vi "parse_file.vi"(0 "File Name With Extension":string) -> (1 "command vector":T1[](array[typedef]), 2 "file_status":string)   [LabVIEW 2014]
uses:
  vi_execute.ctl
panel:
  out "error out":errorcluster
  out "File Contents":string
  out "Lines":string[](array[string])
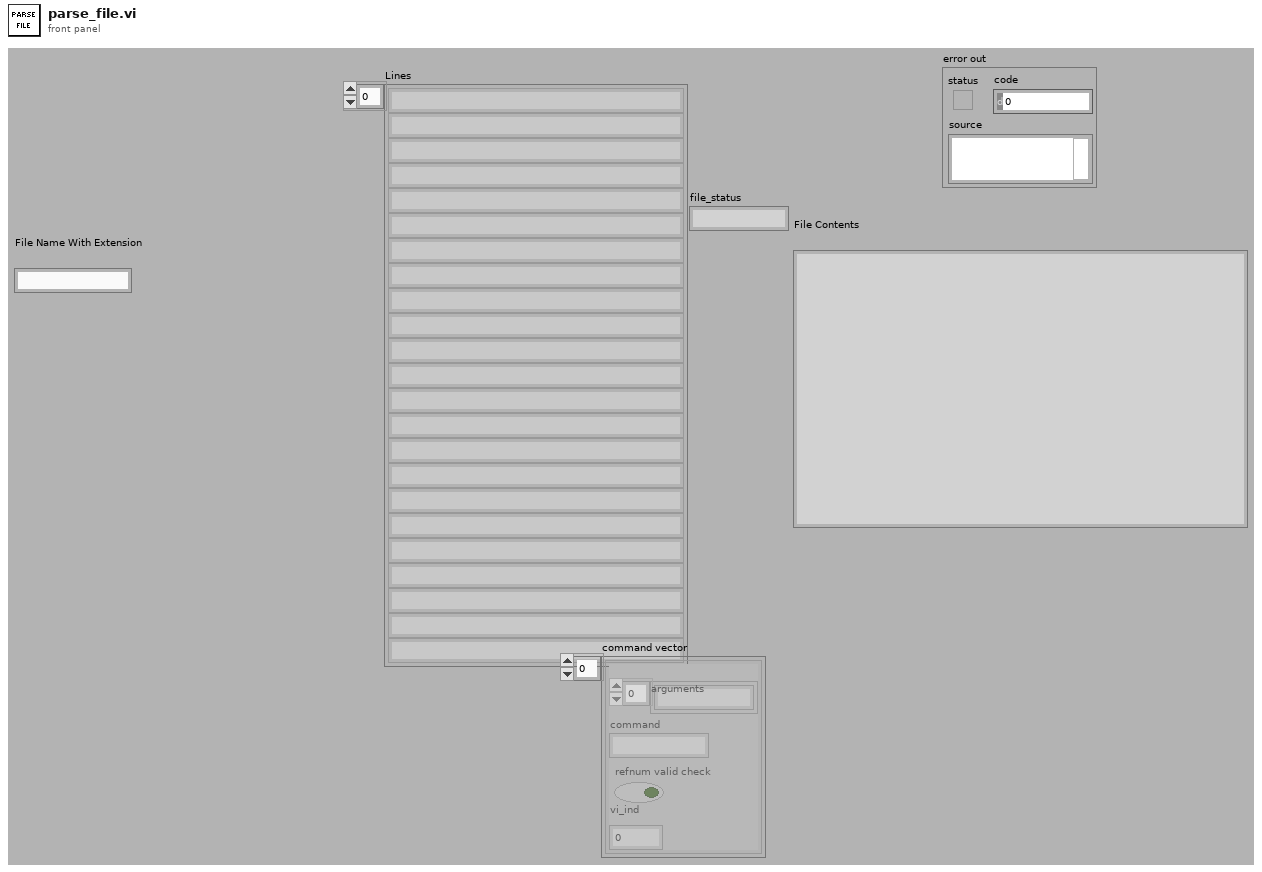
[diagram p1: front panel]
types:
  T1 = typedef "vi_execute.ctl" = cluster{"arguments":string[], "command":string, "refnum valid check":bool, "vi_ind":u8}
  T2 = cluster{"arguments":string[], "refnum name out":string, bool, "index":u8}
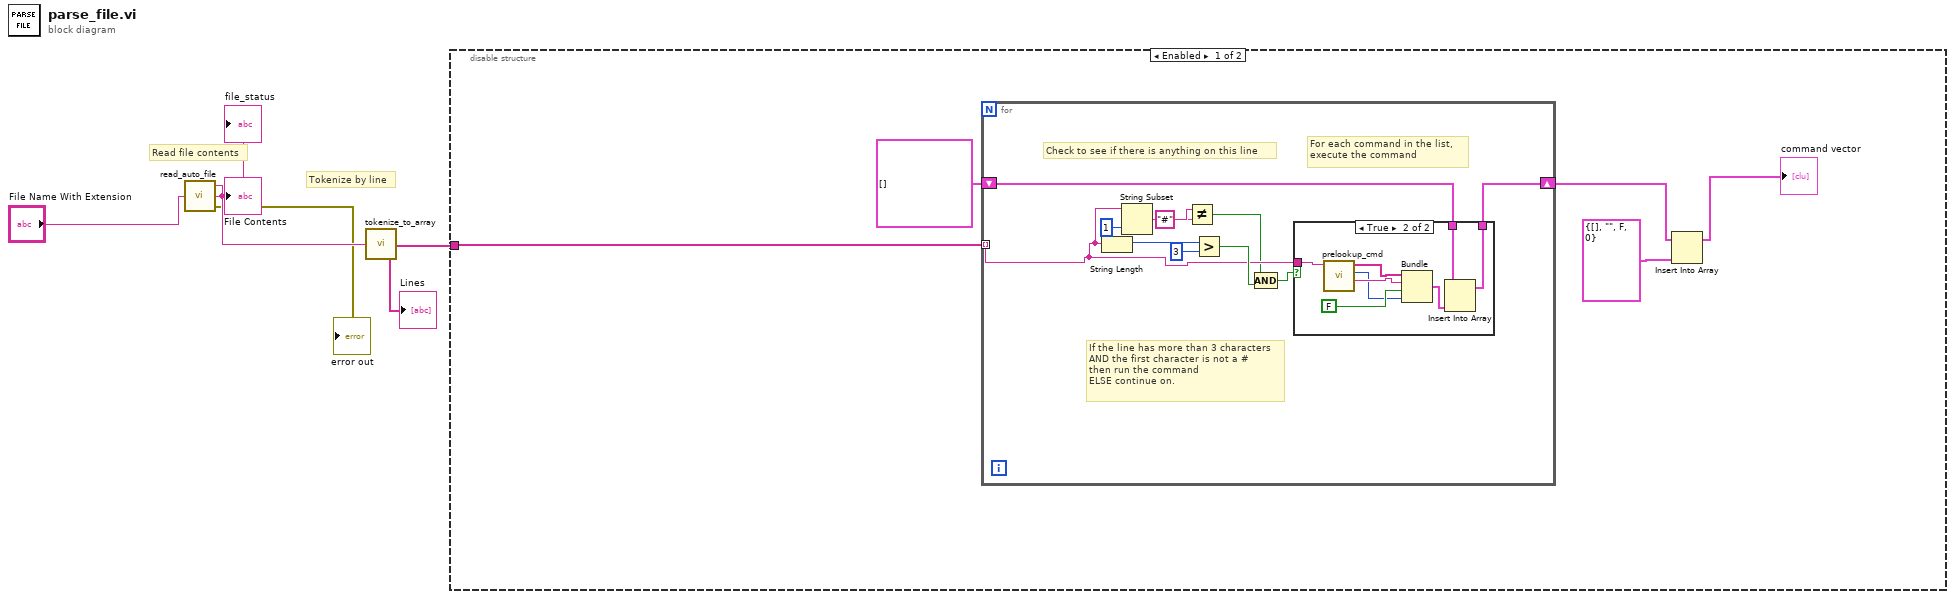
[diagram p0: block diagram]
diagram:
  # "Tokenize by line"
  # "Read file contents"
  n1 = call "read_auto_file.vi"("File Name With Extension"="File Name With Extension") -> ("File Contents"=w5:string, "file_status"=→"file_status":string, "error out"=→"error out":errorcluster)
  "File Contents" <- w5
  n2 = call "tokenize_to_array.vi"("File Contents"=w5) -> ("Lines"=w3:string[])
  "Lines" <- w3
  n3 = disable-structure shown="Enabled" {
    disable-tunnel: w3 -> [w10 _]
    frame Enabled {
      n4 = for {
        tunnel: w10 -> [w17] mode=indexing
        shift-right: [w11] -> w8
        shift-left: T1[] [] -> [w12]
        # "If the line has more than 3 characters\nAND the first character is not a #\nthen run the command\nELSE continue on."
        # "Check to see if there is anything on this line"
        # "For each command in the list,\nexecute the command"
        n5 = String Length(string=w17) -> (length=w21:i32)
        n6 = String Subset(string=w17, length (rest)=1 ("length (rest)")) -> (substring=w15:string)  [unwired: 1 out]
        n7 = Not Equal?(x=w15, y="#") -> (x != y?=w13:bool)
        n8 = Greater?(x=w21, y=3) -> (0:w18:bool)
        n9 = Compound Arithmetic op=AND(w13, w18) -> (w19:bool)
        n10 = case shown="True" w19 {
          tunnel: w17 -> [_ w26]
          tunnel: w12 -> [w22 w28]
          tunnel: [w22 w27] -> w11
          frame False {
          }
          frame True {
            n11 = call "prelookup_cmd.vi"("Command"=w26) -> ("refnum name out"=w25:string, "index"=w23:u8, "arguments"=w30:string[])  [unwired: 8 out]
            n12 = Bundle("arguments"=w30, "refnum name out"=w25, FALSE, "index"=w23) -> (w29:T2)  [unwired: 1 in]
            n13 = Insert Into Array(array=w28, new element=w29) -> (w27:T1[])  [unwired: 1 in]
          }
        }
      }
      n14 = Insert Into Array(array=w8, new element=T1 {"arguments"=[], "command"="", "refnum valid check"=FALSE, "vi_ind"=0} ("new element/subarray")) -> (→"command vector":T1[])  [unwired: 1 in]
    }
    frame Disabled {
    }
  }
